vi "AMI_Merge_Cluster.vi"(1 "AMI_Control":T2, 2 "AMI_Status":T3={"Y-Axis (T)"=0.0, "Z-Axis (T)"=0.0, "B AMI (T)"=0.0, "Phi AMI (Deg) "=0.0, "Switch Heater Y"=FALSE, "Switch Heater Z"=FALSE, "Y Axis Status"=enum."RAMPING", "Z Axis Status"=enum."RAMPING"}) -> (0 "AMI_Cluster":T1={"Y Axis Status"=enum."RAMPING", "Z Axis Status"=enum."RAMPING", "Y-Axis (T)"=0.0, "Y-Axis Setpoint (T)"=0.0, "Y-Axis Rate (T/min)"=0.0, "Z-Axis (T)"=0.0, "Z-Axis Setpoint (T)"=0.0, "Z-Axis Rate (T/min)"=0.0, "B AMI rate (T)"=0.0, "AMI Monitor"=FALSE, "AMI Set field rates"=FALSE, "AMI Set field"=FALSE, "Switch Heater Y"=FALSE, "Switch Heater Z"=FALSE, "Switch Heater"=FALSE, "B AMI (T)"=0.0, "B AMI Setpoint (T)"=0.0, "Phi AMI (Deg) "=0.0, "Phi AMI Setpoint (Deg) "=0.0})   [LabVIEW 2019]
uses:
  AMI/AMI_Status.ctl
  AMI/AMI_Control.ctl
  AMI/AMI_cluster.ctl
panel:
  # "AMI-Cluster"
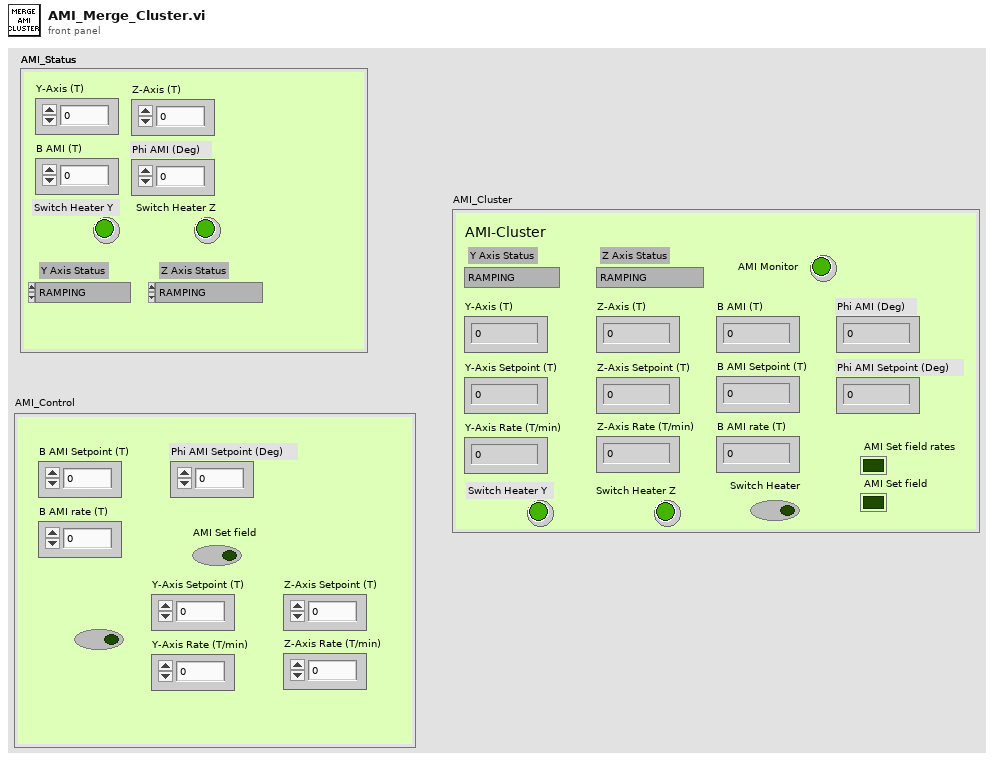
[diagram p1: front panel]
types:
  T1 = typedef "AMI_cluster.ctl" = cluster{"Y Axis Status":enum16{"", "RAMPING", "HOLDING", "PAUSED", "MANUAL UP", "MANUAL DOWN", "ZEROING CURRENT", "QUENCH DETECTED", "HEATING SWITCH", "AT ZER0", "COOLING SWITCH"}, "Z Axis Status":enum16{"", "RAMPING", "HOLDING", "PAUSED", "MANUAL UP", "MANUAL DOWN", "ZEROING CURRENT", "QUENCH DETECTED", "HEATING SWITCH", "AT ZER0", "COOLING SWITCH"}, "Y-Axis (T)":dbl, "Y-Axis Setpoint (T)":dbl, "Y-Axis Rate (T/min)":dbl, "Z-Axis (T)":dbl, "Z-Axis Setpoint (T)":dbl, "Z-Axis Rate (T/min)":dbl, "B AMI rate (T)":dbl, "AMI Monitor":bool, "AMI Set field rates":bool, "AMI Set field":bool, "Switch Heater Y":bool, "Switch Heater Z":bool, "Switch Heater":bool, "B AMI (T)":dbl, "B AMI Setpoint (T)":dbl, "Phi AMI (Deg) ":dbl, "Phi AMI Setpoint (Deg) ":dbl}
  T2 = typedef "AMI_Control.ctl" = cluster{"B AMI rate (T)":dbl, "AMI Set field":bool, "B AMI Setpoint (T)":dbl, "Phi AMI Setpoint (Deg) ":dbl, "Switch Heater":bool, "Y-Axis Setpoint (T)":dbl, "Y-Axis Rate (T/min)":dbl, "Z-Axis Setpoint (T)":dbl, "Z-Axis Rate (T/min)":dbl}
  T3 = typedef "AMI_Status.ctl" = cluster{"Y-Axis (T)":dbl, "Z-Axis (T)":dbl, "B AMI (T)":dbl, "Phi AMI (Deg) ":dbl, "Switch Heater Y":bool, "Switch Heater Z":bool, "Y Axis Status":enum16{"", "RAMPING", "HOLDING", "PAUSED", "MANUAL UP", "MANUAL DOWN", "ZEROING CURRENT", "QUENCH DETECTED", "HEATING SWITCH", "AT ZER0", "COOLING SWITCH"}, "Z Axis Status":enum16{"", "RAMPING", "HOLDING", "PAUSED", "MANUAL UP", "MANUAL DOWN", "ZEROING CURRENT", "QUENCH DETECTED", "HEATING SWITCH", "AT ZER0", "COOLING SWITCH"}}
  T4 = enum16{"", "RAMPING", "HOLDING", "PAUSED", "MANUAL UP", "MANUAL DOWN", "ZEROING CURRENT", "QUENCH DETECTED", "HEATING SWITCH", "AT ZER0", "COOLING SWITCH"}
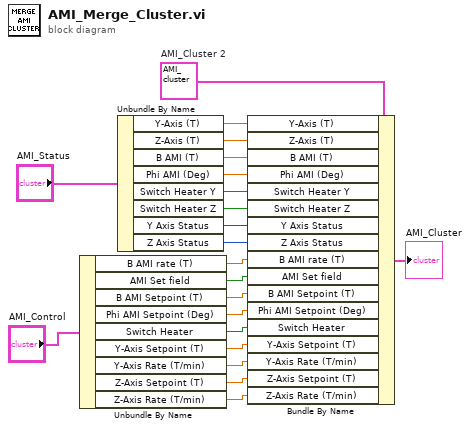
[diagram p0: block diagram]
diagram:
  w19 = T1 {"Y Axis Status"=enum."RAMPING", "Z Axis Status"=enum."RAMPING", "Y-Axis (T)"=0.0, "Y-Axis Setpoint (T)"=0.0, "Y-Axis Rate (T/min)"=0.0, "Z-Axis (T)"=0.0, "Z-Axis Setpoint (T)"=0.0, "Z-Axis Rate (T/min)"=0.0, "B AMI rate (T)"=0.0, "AMI Monitor"=FALSE, "AMI Set field rates"=FALSE, "AMI Set field"=FALSE, "Switch Heater Y"=FALSE, "Switch Heater Z"=FALSE, "Switch Heater"=FALSE, "B AMI (T)"=0.0, "B AMI Setpoint (T)"=0.0, "Phi AMI (Deg) "=0.0, "Phi AMI Setpoint (Deg) "=0.0}  # AMI_Cluster 2
  n1 = Unbundle By Name("AMI_Control") -> ("B AMI rate (T)"=w9:dbl, "AMI Set field"=w8:bool, "B AMI Setpoint (T)"=w7:dbl, "Phi AMI Setpoint (Deg)"=w6:dbl, "Switch Heater"=w4:bool, "Y-Axis Setpoint (T)"=w5:dbl, "Y-Axis Rate (T/min)"=w3:dbl, "Z-Axis Setpoint (T)"=w2:dbl, "Z-Axis Rate (T/min)"=w1:dbl)
  n2 = Unbundle By Name("AMI_Status") -> ("Y-Axis (T)"=w17:dbl, "Z-Axis (T)"=w16:dbl, "B AMI (T)"=w15:dbl, "Phi AMI (Deg)"=w14:dbl, "Switch Heater Y"=w13:bool, "Switch Heater Z"=w12:bool, "Y Axis Status"=w11:T4, "Z Axis Status"=w10:T4)
  n3 = Bundle By Name(cluster=w19, "Y-Axis (T)"=w17, "Z-Axis (T)"=w16, "B AMI (T)"=w15, "Phi AMI (Deg)"=w14, "Switch Heater Y"=w13, "Switch Heater Z"=w12, "Y Axis Status"=w11, "Z Axis Status"=w10, "B AMI rate (T)"=w9, "AMI Set field"=w8, "B AMI Setpoint (T)"=w7, "Phi AMI Setpoint (Deg)"=w6, "Switch Heater"=w4, "Y-Axis Setpoint (T)"=w5, "Y-Axis Rate (T/min)"=w3, "Z-Axis Setpoint (T)"=w2, "Z-Axis Rate (T/min)"=w1) -> (→"AMI_Cluster":T1)
